vi "Cmd Create Parameters.vi"(4 "error in (no error)":errorcluster, 5 "parameters":T1[](array[typedef]), 6 "ADODB.Parameters":refnum<k7>, 7 "ADODB._Command":refnum<k7>) -> (0 "error out":errorcluster, 2 "ADODB.Parameters out":refnum<k7>, 3 "ADODB._Command out":refnum<k7>)   [LabVIEW 2020, in "NI_Database_API.lvlib"]
doc: "Creates the parameters defined by the information contained in the array for the database connection defined by the command and parameter refnums."
uses:
  <vilib>/addons/database/NI_Database_API.lvlib
  <vilib>/addons/database/Auxilliary.llb/DB Tools Parameter Info.ctl
  <vilib>/addons/database/Auxilliary.llb/DB Tools DataTypes.ctl
  <vilib>/addons/database/Auxilliary.llb/DB Tools Parameter Dir.ctl
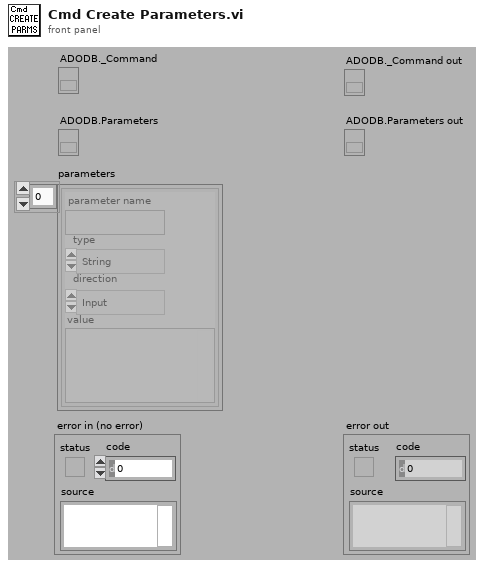
[diagram p1: front panel]
types:
  T1 = typedef "NI_Database_API.lvlib/DB Tools Parameter Info.ctl" = cluster{"parameter name":string, "type":T2, "direction":T3, "value":variant}
  T2 = typedef "NI_Database_API.lvlib/DB Tools DataTypes.ctl" = enum16{"String", "Long (I32)", "Single (SGL)", "Double (DBL)", "Date/Time", "Binary"}
  T3 = typedef "NI_Database_API.lvlib/DB Tools Parameter Dir.ctl" = enum32{"Input", "Output", "Input/Output", "Return Value"}
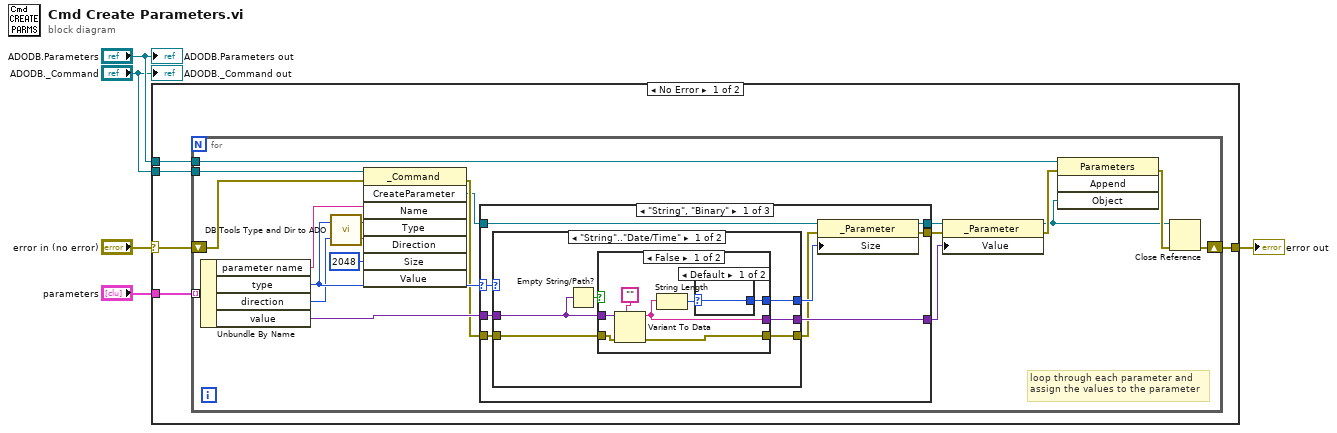
[diagram p0: block diagram]
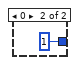
[diagram p2: hidden frame]
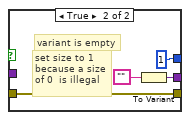
[diagram p3: hidden frame]
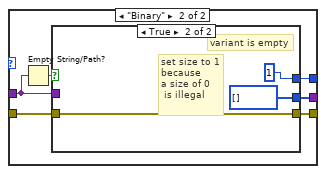
[diagram p4: hidden frame]
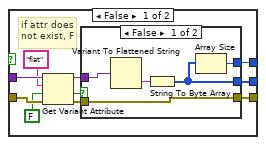
[diagram p5: hidden frame]
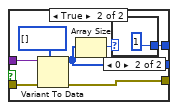
[diagram p6: hidden frame]
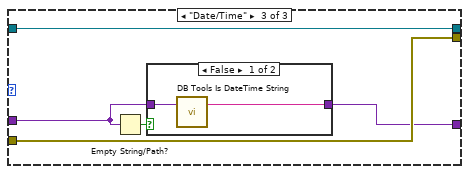
[diagram p9: hidden frame]
diagram:
  n1 = case shown="No Error" "error in (no error)" {
    selector: "error in (no error)" -> [w6 w103]
    tunnel: "ADODB.Parameters" -> [w10 _]
    tunnel: "ADODB._Command" -> [w9 _]
    tunnel: [w8 w103] -> w5
    tunnel: "parameters" -> [w7 _]
    frame No Error {
      n2 = for {
        tunnel: w9 -> [w18]
        tunnel: w10 -> [w30]
        shift-right: [w28] -> w8
        shift-left: w6 -> [w17]
        tunnel: w7 -> [w27] mode=indexing
        # "loop through each parameter and\nassign the values to the parameter"
        n3 = Unbundle By Name(w27) -> ("parameter name"=w16:string, "type"=w23:T2, "direction"=w22:T3, "value"=w26:variant)
        n4 = call <vilib>:"DB Tools Type and Dir to ADO.vi"("direction"=w22, "data type"=w23) -> ("ADO direction"=w14:u16, "ADO type"=w15:u16)
        n5 = invoke class="_Command" method="CreateParameter"(reference=w18, error in=w17, "Name"=w16, "Type"=w15, "Direction"=w14, "Size"=2048) -> (error out=w13:errorcluster, "CreateParameter"=w12:refnum<k7>)  [unwired: 2 in, 6 out]
        n6 = case shown="\"String\", \"Binary\"" w23 {
          selector: w23 -> [w35 _ _]
          tunnel: w26 -> [w34 w92 w95]
          tunnel: [w39 w94 w99] -> w25
          tunnel: [w38 w93 w98] -> w24
          tunnel: w12 -> [w37 w94 w99]
          tunnel: w13 -> [w33 w93 w98]
          tunnel: [w32 w92 w97] -> w19
          frame "String", "Binary" {
            n7 = case shown="\"String\"..\"Date/Time\"" w35 {
              tunnel: [w44 w63] -> w36
              tunnel: w34 -> [w43 w60]
              tunnel: w33 -> [w42 w59]
              tunnel: [w41 w62] -> w31
              tunnel: [w40 w61] -> w32
              frame "String".."Date/Time" {
                n8 = Empty String/Path?(string/path=w43) -> (empty?=w45:bool)
                n9 = case shown="False" w45 {
                  tunnel: [w51 1] -> w44
                  tunnel: w43 -> [w50 _]
                  tunnel: w42 -> [w49 w57]
                  tunnel: [w48 w57] -> w41
                  tunnel: [w46 w55] -> w40
                  frame False {
                    n10 = Variant To Data(error in=w49, type="", Variant=w50) -> (data=w46:string, error out=w48:errorcluster)
                    n11 = String Length(string=w46) -> (length=w52:i32)
                    n12 = case shown="Default" w52 {
                      selector: w52 -> [w53 _]
                      tunnel: [w53 1] -> w51
                      frame Default {
                      }
                      frame 0 {
                      }
                    }
                  }
                  frame True {
                    # "set size to 1 \nbecause a size \nof 0  is illegal"
                    # "variant is empty"
                    n13 = To Variant(anything="") -> (Variant=w55:variant)
                  }
                }
              }
              frame "Binary" {
                n14 = Empty String/Path?(string/path=w60) -> (empty?=w64:bool)
                n15 = case shown="True" w64 {
                  tunnel: [w73 1] -> w63
                  tunnel: w59 -> [w70 w90]
                  tunnel: [w74 w90] -> w62
                  tunnel: [w72 u8[] [] ("Array Constant")] -> w61
                  tunnel: w60 -> [w71 _]
                  frame False {
                    # "if attr does\nnot exist, F"
                    n16 = Get Variant Attribute(Variant=w71, name="flat", default value (empty Variant)=FALSE, error in=w70) -> (duplicate Variant=w65:variant, value=w67:bool, error out=w66:errorcluster)  [unwired: 1 out]
                    n17 = case shown="False" w67 {
                      tunnel: [w75 w86] -> w74
                      tunnel: [w76 w81] -> w73
                      tunnel: [w77 w84] -> w72
                      tunnel: w65 -> [w79 w83]
                      tunnel: w66 -> [w75 w82]
                      frame False {
                        n18 = Variant To Flattened String(Variant=w79) -> (data string=w78:string)  [unwired: 1 out]
                        n19 = String To Byte Array(string=w78) -> (unsigned byte array=w77:u8[])
                        n20 = Array Size(array=w77) -> (size(s)=w76:i32)
                      }
                      frame True {
                        n21 = Variant To Data(error in=w82, type=u8[] [] ("Array Constant"), Variant=w83) -> (data=w84:u8[], error out=w86:errorcluster)
                        n22 = Array Size(array=w84) -> (size(s)=w80:i32)
                        n23 = case shown="0" w80 {
                          selector: w80 -> [w87 _]
                          tunnel: [w87 1] -> w81
                          frame Default {
                          }
                          frame 0 {
                          }
                        }
                      }
                    }
                  }
                  frame True {
                    # "set size to 1 \nbecause\na size of 0\n is illegal"
                    # "variant is empty"
                  }
                }
              }
            }
            n24 = property class="_Parameter"(reference=w37, error in=w31, "Size"=w36) -> (reference out=w39:refnum<k7>, error out=w38:errorcluster)
          }
          frame "Long (I32)".."Double (DBL)" {
          }
          frame "Date/Time" {
            n25 = Empty String/Path?(string/path=w95) -> (empty?=w96:bool)
            n26 = case shown="False" w96 {
              tunnel: [w100 w102] -> w97
              tunnel: w95 -> [w101 w102]
              frame False {
                n27 = call <vilib>:"DB Tools Is DateTime String.vi"("string or date/time"=w101) -> ("data"=w100:string)  [unwired: 1 in, 1 out]
              }
              frame True {
              }
            }
          }
        }
        n28 = property class="_Parameter"(reference=w25, error in=w24, "Value"=w19) -> (reference out=w20:refnum<k7>, error out=w21:errorcluster)
        n29 = invoke class="Parameters" method="Append"(reference=w30, error in=w21, "Object"=w20) -> (error out=w29:errorcluster)  [unwired: 1 in, 3 out]
        n30 = Close Reference(reference=w20, error in (no error)=w29) -> (error out=w28:errorcluster)
      }
    }
    frame Error {
    }
  }
  "error out" <- w5
  "ADODB._Command out" <- "ADODB._Command"
  "ADODB.Parameters out" <- "ADODB.Parameters"
